vi "SavePars.vi"() -> (0 "Error":bool=TRUE)   [LabVIEW 2014]
uses:
  globals/AzCamGlobals.vi
panel:
  out "Error":bool
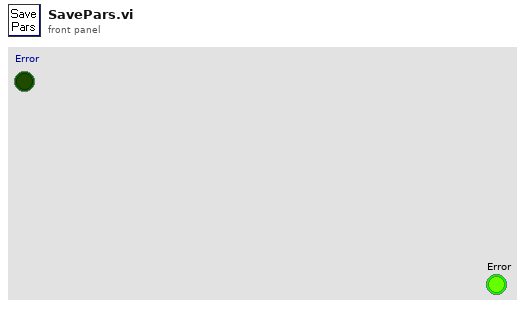
[diagram p1: front panel]
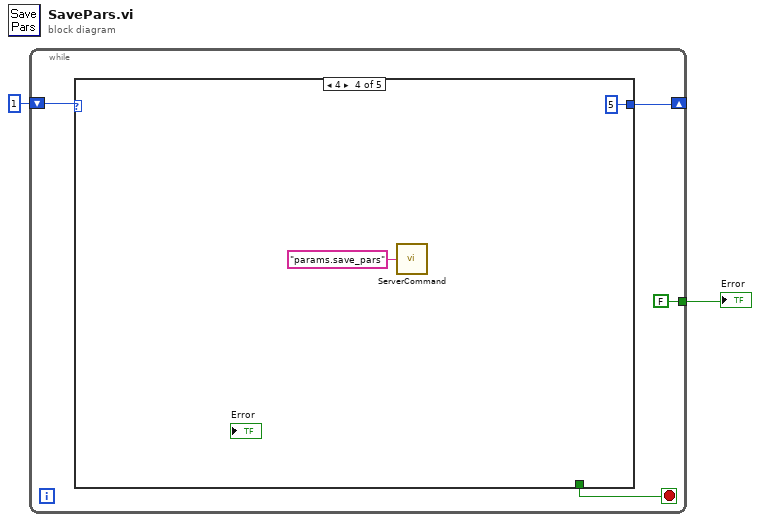
[diagram p0: block diagram]
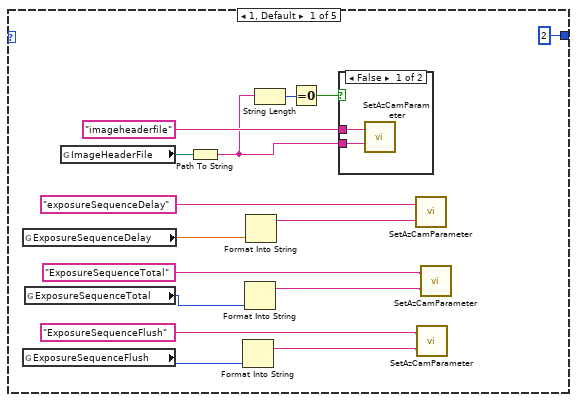
[diagram p2: hidden frame]
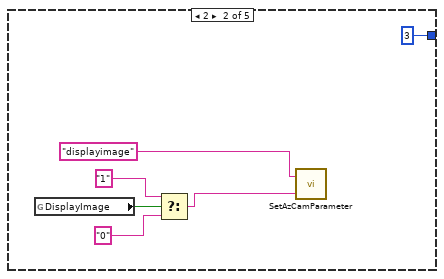
[diagram p4: hidden frame]
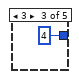
[diagram p5: hidden frame]
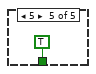
[diagram p6: hidden frame]
diagram:
  n1 = while {
    shift-right: [w6] -> _
    shift-left: 1 -> [w5]
    tunnel: [FALSE ("Error")] -> w1
    stop <- w4 stop-if-true
    n2 = case shown="4" w5 {
      tunnel: [2 3 4 5 _] -> w6
      tunnel: [_ _ _ _ TRUE ("status")] -> w4
      frame 1, Default {
        n3 = global read "AzCamGlobals.vi" "ExposureSequenceDelay"() -> (w19:dbl)
        n4 = global read "AzCamGlobals.vi" "ExposureSequenceFlush"() -> (w17:i32)
        n5 = global read "AzCamGlobals.vi" "ExposureSequenceTotal"() -> (w18:i32)
        n6 = global read "AzCamGlobals.vi" "ImageHeaderFile"() -> (w20:path)
        n7 = Path To String(path=w20) -> (string=w13:string)
        n8 = Format Into String(w17) -> (resulting string=w7:string)  [unwired: 3 in, 1 out]
        n9 = Format Into String(w18) -> (resulting string=w9:string)  [unwired: 3 in, 1 out]
        n10 = Format Into String(w19) -> (resulting string=w11:string)  [unwired: 3 in, 1 out]
        n11 = String Length(string=w13) -> (length=w15:i32)
        n12 = Equal To 0?(x=w15) -> (x = 0?=w14:bool)
        n13 = case shown="False" w14 {
          tunnel: w13 -> [w23 _]
          tunnel: "imageheaderfile" ("Parameter") -> [w22 _]
          frame False {
            n14 = call "SetAzCamParameter.vi"("Value"=w23, "Parameter"=w22) -> ()  [unwired: 1 out]
          }
          frame True {
          }
        }
        n15 = call "SetAzCamParameter.vi"("Value"=w11, "Parameter"="exposureSequenceDelay") -> ()  [unwired: 1 out]
        n16 = call "SetAzCamParameter.vi"("Value"=w7, "Parameter"="ExposureSequenceFlush") -> ()  [unwired: 1 out]
        n17 = call "SetAzCamParameter.vi"("Value"=w9, "Parameter"="ExposureSequenceTotal") -> ()  [unwired: 1 out]
      }
      frame 2 {
        n18 = global read "AzCamGlobals.vi" "DisplayImage"() -> (w24:bool)
        n19 = Select(t="1" ("y"), s=w24, f="0" ("y")) -> (s? t:f=w28:string)
        n20 = call "SetAzCamParameter.vi"("Value"=w28, "Parameter"="displayimage" ("key")) -> ()  [unwired: 1 out]
      }
      frame 3 {
      }
      frame 4 {
        n21 = call "ServerCommand.vi"("Command"="params.save_pars") -> ()  [unwired: 2 out]
      }
      frame 5 {
      }
    }
  }
  "Error" <- w1
